vi "Graph Scale Axis.vi"(8 "error in":errorcluster, 11 "Values":dbl[](array[numeric])) -> (0 "error out":errorcluster, 2 "Minumum":dbl, 3 "Maximum":dbl)   [LabVIEW 2014, in "hse-misc.lvlib"]
doc: "Calculates usefull values for the Graph scaling (Minimum, Maximum) that go 10% over the min/max-values and include zero."
uses:
  hse-misc.lvlib
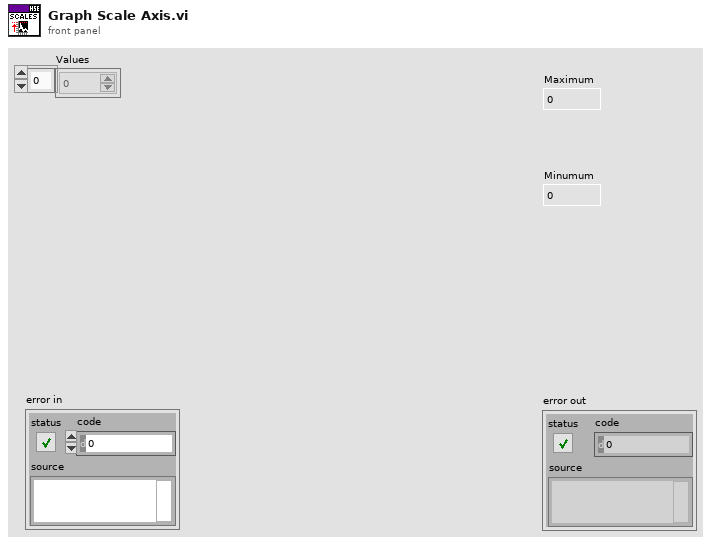
[diagram p1: front panel]
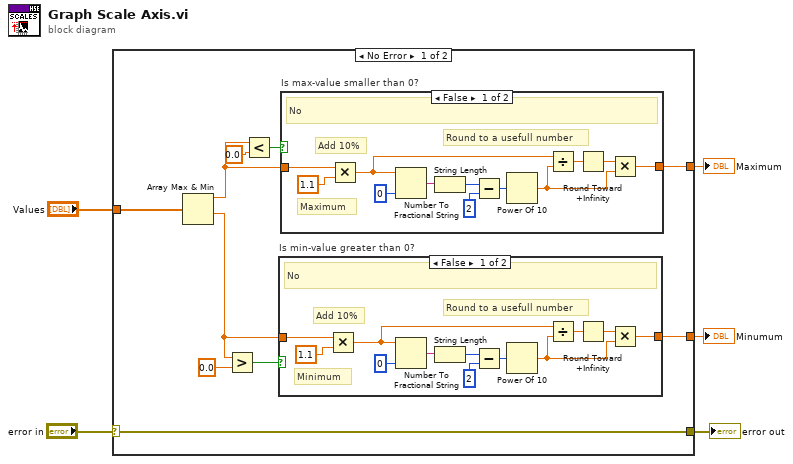
[diagram p0: block diagram]
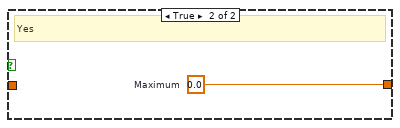
[diagram p2: hidden frame]
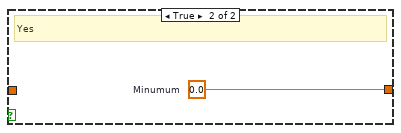
[diagram p3: hidden frame]
diagram:
  n1 = case shown="No Error" "error in" {
    selector: "error in" -> [w15 w42]
    tunnel: [w15 w42] -> w4
    tunnel: "Values" -> [w14 _]
    tunnel: [w7 _] -> w2
    tunnel: [w6 _] -> w1
    frame No Error {
      n2 = Array Max & Min(array=w14) -> (max value=w9:dbl, min value=w11:dbl)  [unwired: 2 out]
      n3 = Greater?(x=w11, y=0.0) -> (0:w12:bool)
      n4 = Less?(x=w9, y=0.0) -> (x < y?=w10:bool)
      n5 = case "Is min-value greater than 0?" shown="False" w12 {
        tunnel: [w29 w41] -> w6
        tunnel: w11 -> [w40 _]
        frame False {
          # "Round to a usefull number"
          # "Minimum"
          # "Add 10%"
          # "No"
          n6 = Multiply(x=w40, y=1.1) -> (x*y=w30:dbl)
          n7 = Number To Fractional String(number=w30, precision (6)=i16 0) -> (F-format string=w32:string)  [unwired: 2 in]
          n8 = String Length(string=w32) -> (length=w33:i32)
          n9 = Subtract(x=w33, y=2) -> (x-y=w35:i32)
          n10 = Power Of 10(x=w35) -> (10^x=w38:dbl)
          n11 = Divide(x=w30, y=w38) -> (x/y=w36:dbl)
          n12 = Round Toward +Infinity(x=w36) -> (ceil(x): smallest int >= x=w37:dbl)
          n13 = Multiply(x=w37, y=w38) -> (x*y=w29:dbl)
        }
        frame True {
          w41 = 0.0  # Minumum
          # "Yes"
        }
      }
      n14 = case "Is max-value smaller than 0?" shown="False" w10 {
        tunnel: [w16 w28] -> w7
        tunnel: w9 -> [w27 _]
        frame False {
          # "Round to a usefull number"
          # "Maximum"
          # "Add 10%"
          # "No"
          n15 = Multiply(x=w27, y=1.1) -> (x*y=w17:dbl)
          n16 = Number To Fractional String(number=w17, precision (6)=i16 0) -> (F-format string=w19:string)  [unwired: 2 in]
          n17 = String Length(string=w19) -> (length=w20:i32)
          n18 = Subtract(x=w20, y=2) -> (x-y=w22:i32)
          n19 = Power Of 10(x=w22) -> (10^x=w25:dbl)
          n20 = Divide(x=w17, y=w25) -> (x/y=w23:dbl)
          n21 = Round Toward +Infinity(x=w23) -> (ceil(x): smallest int >= x=w24:dbl)
          n22 = Multiply(x=w24, y=w25) -> (x*y=w16:dbl)
        }
        frame True {
          w28 = 0.0  # Maximum
          # "Yes"
        }
      }
    }
    frame Error {
    }
  }
  "error out" <- w4
  "Maximum" <- w2
  "Minumum" <- w1
